vi "Cluster names.vi"(10 "Name":string, 11 "variant 2":variant) -> (0 "Array":variant[](array[variant]), 1 "Array 2":string[](array[string]), 2 "VCluster":variant, 3 "String":string)   [LabVIEW 2013]
uses:
  subVis/ROI_TypDef.ctl
  shared/OnOffTypeDef.ctl
  <vilib>/vision/Image Controls.llb/IMAQ Image.ctl
  <vilib>/userdefined/High Color/IMAQdx.ctl
  subVis/CamAtributes_TypDEfTestDevice.ctl
  subVis/TriggerModeString_TypDEf.ctl
  shared/numericVariable_TypeDef.ctl
  BaseDriver/BaseDriver.lvclass
panel:
  in  "Cluster of class private data":T7
  out "Data Name":string
  out "Array of VData":variant[](array[variant])
  in  "error in (no error)":errorcluster
  out "data out":string[][](array[string])
  in  "data in":string[][](array[string])=[["name", "value", "min", "max", "stepsize", "units", "variabletype", "tolerance", "valueactual"], ["Position.Axis 111", "0.000000000000000", "-999999", "999999", "0.000000000000000", "", "numeric", "0.000000000000000", "0.000000000000000"], ["Position.Axis 112", "0.000000000000000", "-999999", "999999", "0.000000000000000", "", "numeric", "0.000000000000000", "0.000000000000000"], ["Position.Axis 113", "0.000000000000000", "-999999", "999999", "0.000000000000000", "", "numeric", "0.000000000000000", "0.000000000000000"], ["Position.Axis 121", "0.000000000000000", "-999999", "999999", "0.000000000000000", "", "numeric", "0.000000000000000", "0.000000000000000"], ["Position.Axis 122", "0.000000000000000", "-999999", "999999", "0.000000000000000", "", "numeric", "0.000000000000000", "0.000000000000000"], ["Position.Axis 123", "0.000000000000000", "-999999", "999999", "0.000000000000000", "", "numeric", "0.000000000000000", "0.000000000000000"], ["Position.Axis 131", "0.000000000000000", "-999999", "999999", "0.000000000000000", "", "numeric", "0.000000000000000", "0.000000000000000"], ["Position.Axis 132", "0.000000000000000", "-999999", "999999", "0.000000000000000", "", "numeric", "0.000000000000000", "0.000000000000000"], ["Position.Axis 133", "0.000000000000000", "-999999", "999999", "0.000000000000000", "", "numeric", "0.000000000000000", "0.000000000000000"], ["Position.Axis 141", "0.000000000000000", "-999999", "999999", "0.000000000000000", "", "numeric", "0.000000000000000", "0.000000000000000"], ["Position.Axis 142", "0.000000000000000", "-999999", "999999", "0.000000000000000", "", "numeric", "0.000000000000000", "0.000000000000000"], ["Position.Axis 143", "0.000000000000000", "-999999", "999999", "0.000000000000000", "", "numeric", "0.000000000000000", "0.000000000000000"], ["Position.Axis 231", "0.000000000000000", "-999999", "999999", "0.000000000000000", "", "numeric", "0.000000000000000", "0.000000000000000"], ["Position.Axis 232", "0.000000000000000", "-999999", "-999999", "0.000000000000000", "", "numeric", "0.000000000000000", "0.000000000000000"], ["Position.Axis 233", "0.000000000000000", "-999999", "999999", "0.000000000000000", "", "numeric", "0.000000000000000", "0.000000000000000"], ["Position.Axis 241", "0.000000000000000", "-999999", "999999", "0.000000000000000", "", "numeric", "0.000000000000000", "0.000000000000000"], ["Position.Axis 242", "0.000000000000000", "-999999", "999999", "0.000000000000000", "", "numeric", "0.000000000000000", "0.000000000000000"], ["Position.Axis 243", "0.000000000000000", "-999999", "999999", "0.000000000000000", "", "numeric", "0.000000000000000", "0.000000000000000"], ["Position.Axis 311", "0.000000000000000", "-999999", "999999", "0.000000000000000", "", "numeric", "0.000000000000000", "0.000000000000000"], ["Position.Axis 312", "0.000000000000000", "-999999", "999999", "0.000000000000000", "", "numeric", "0.000000000000000", "0.000000000000000"], ["Position.Axis 321", "0.000000000000000", "-999999", "999999", "0.000000000000000", "", "numeric", "0.000000000000000", "0.000000000000000"], ["Position.Axis 322", "0.000000000000000", "-999999", "999999", "0.000000000000000", "", "numeric", "0.000000000000000", "0.000000000000000"], ["Position.Axis 323", "0.000000000000000", "-999999", "999999", "0.000000000000000", "", "numeric", "0.000000000000000", "0.000000000000000"], ["Position.Axis 331", "0.000000000000000", "-999999", "999999", "0.000000000000000", "", "numeric", "0.000000000000000", "0.000000000000000"], ["Position.Axis 332", "0.000000000000000", "-999999", "0.00000000000999999", "0.000000000000000", "", "numeric", "0.000000000000000", "0.000000000000000"], ["Position.Axis 333", "0.000000000000000", "-999999", "999999", "0.000000000000000", "", "numeric", "0.000000000000000", "0.000000000000000"], ["Position.Axis 341", "0.000000000000000", "-999999", "9999990000", "0.000000000000000", "", "numeric", "0.000000000000000", "0.000000000000000"], ["Position.Axis 342", "0.000000000000000", "-999999", "999999", "0.000000000000000", "", "numeric", "0.000000000000000", "0.000000000000000"], ["Position.Axis 343", "0.000000000000000", "-999999", "999999", "0.000000000000000", "", "numeric", "0.000000000000000", "0.000000000000000"], ["Position.Axis 411", "0.000000000000000", "-999999", "999999", "0.000000000000000", "", "numeric", "0.000000000000000", "0.000000000000000"], ["Position.Axis 412", "0.000000000000000", "-999999", "999999", "0.000000000000000", "", "numeric", "0.000000000000000", "0.000000000000000"], ["Position.Axis 413", "0.000000000000000", "-999999", "999999", "0.000000000000000", "", "numeric", "0.000000000000000", "0.000000000000000"], ["Position.Axis 421", "0.000000000000000", "-999999", "999999", "0.000000000000000", "", "numeric", "0.000000000000000", "0.000000000000000"], ["Position.Axis 422", "0.000000000000000", "-999999", "999999", "0.000000000000000", "", "numeric", "0.000000000000000", "0.000000000000000"], ["Position.Axis 423", "0.000000000000000", "-999999", "999999", "0.000000000000000", "", "numeric", "0.000000000000000", "0.000000000000000"], ["Position.Axis 431", "0.000000000000000", "-999999", "999999", "0.000000000000000", "", "numeric", "0.000000000000000", "0.000000000000000"], ["Position.Axis 432", "0.000000000000000", "-99999900000", "999999", "0.000000000000000", "", "numeric", "0.000000000000000", "0.000000000000000"], ["Position.Axis 433", "0.000000000000000", "-999999", "999999", "0.000000000000000", "", "numeric", "0.000000000000000", "0.000000000000000"], ["Position.Axis 441", "0.000000000000000", "-999999", "999999", "0.000000000000000", "", "numeric", "0.000000000000000", "0.000000000000000"], ["Position.Axis 442", "0.000000000000000", "-999999", "999999", "0.000000000000000", "", "numeric", "0.000000000000000", "0.000000000000000"], ["Position.Axis 443", "0.000000000000000", "-999999", "999999", "0.000000000000000", "", "numeric", "0.000000000000000", "0.000000000000000"], ["Position.Axis 511", "0.000000000000000", "-999999", "999999", "0.000000000000000", "", "numeric", "0.000000000000000", "0.000000000000000"], ["Position.Axis 512", "0.000000000000000", "-999999", "999999", "0.000000000000000", "", "numeric", "0.000000000000000", "0.000000000000000"], ["Position.Axis 513", "0.000000000000000", "-999999", "999999", "0.000000000000000", "", "numeric", "0.000000000000000", "0.000000000000000"], ["Position.Axis 521", "0.000000000000000", "-999999", "999999", "0.000000000000000", "", "numeric", "0.000000000000000", "0.000000000000000"], ["Position.Axis 522", "0.000000000000000", "-999999", "999999", "0.000000000000000", "", "numeric", "0.000000000000000", "0.000000000000000"], ["Position.Axis 523", "0.000000000000000", "-999999", "999999", "0.000000000000000", "", "numeric", "0.000000000000000", "0.000000000000000"], ["Position.Axis 531", "0.000000000000000", "-999999", "999999", "0.000000000000000", "", "numeric", "0.000000000000000", "0.000000000000000"], ["Position.Axis 532", "0.000000000000000", "-999999", "999999", "0.000000000000000", "", "numeric", "0.000000000000000", "0.000000000000000"], ["Position.Axis 533", "0.000000000000000", "-999999", "999999", "0.000000000000000", "", "numeric", "0.000000000000000", "0.000000000000000"], ["Position.Axis 541", "0.000000000000000", "-999999", "999999", "0.000000000000000", "", "numeric", "0.000000000000000", "0.000000000000000"], ["Position.Axis 542", "0.000000000000000", "-999999", "999999", "0.000000000000000", "", "numeric", "0.000000000000000", "0.000000000000000"], ["Position.Axis 543", "0.000000000000000", "-999999", "999999", "0.000000000000000", "", "numeric", "0.000000000000000", "0.000000000000000"], ["StepSize.Axis 111", "50", "0", "20000", "0.000000000000000", "", "numeric", "0.000000000000000", "0.000000000000000"], ["StepSize.Axis 112", "50", "0", "20000", "0.000000000000000", "", "numeric", "0.000000000000000", "0.000000000000000"], ["StepSize.Axis 113", "50", "0", "20000", "0.000000000000000", "", "numeric", "0.000000000000000", "0.000000000000000"], ["StepSize.Axis 121", "50", "0", "20000", "0.000000000000000", "", "numeric", "0.000000000000000", "0.000000000000000"], ["StepSize.Axis 122", "50", "0", "20000", "0.000000000000000", "", "numeric", "0.000000000000000", "0.000000000000000"], ["StepSize.Axis 123", "50", "0", "20000", "0.000000000000000", "", "numeric", "0.000000000000000", "0.000000000000000"], ["StepSize.Axis 131", "50", "0", "20000", "0.000000000000000", "", "numeric", "0.000000000000000", "0.000000000000000"], ["StepSize.Axis 132", "50", "0", "20000", "0.000000000000000", "", "numeric", "0.000000000000000", "0.000000000000000"], ["StepSize.Axis 133", "50", "0", "20000", "0.000000000000000", "", "numeric", "0.000000000000000", "0.000000000000000"], ["StepSize.Axis 141", "50", "0", "20000", "0.000000000000000", "", "numeric", "0.000000000000000", "0.000000000000000"], ["StepSize.Axis 142", "50", "0", "20000", "0.000000000000000", "", "numeric", "0.000000000000000", "0.000000000000000"], ["StepSize.Axis 143", "50", "0", "20000", "0.000000000000000", "", "numeric", "0.000000000000000", "0.000000000000000"], ["StepSize.Axis 211", "50", "0", "20000", "0.000000000000000", "", "numeric", "0.000000000000000", "0.000000000000000"], ["StepSize.Axis 212", "50", "0", "20000", "0.000000000000000", "", "numeric", "0.000000000000000", "0.000000000000000"], ["StepSize.Axis 213", "50", "0", "20000", "0.000000000000000", "", "numeric", "0.000000000000000", "0.000000000000000"], ["StepSize.Axis 231", "50", "0", "20000", "0.000000000000000", "", "numeric", "0.000000000000000", "0.000000000000000"], ["StepSize.Axis 232", "50", "0", "20000", "0.000000000000000", "", "numeric", "0.000000000000000", "0.000000000000000"], ["StepSize.Axis 233", "50", "0", "20000", "0.000000000000000", "", "numeric", "0.000000000000000", "0.000000000000000"], ["StepSize.Axis 241", "0", "0", "20000", "0.000000000000000", "", "numeric", "0.000000000000000", "0.000000000000000"], ["StepSize.Axis 242", "50", "0", "20000", "0.000000000000000", "", "numeric", "0.000000000000000", "0.000000000000000"], ["StepSize.Axis 243", "50", "0", "20000", "0.000000000000000", "", "numeric", "0.000000000000000", "0.000000000000000"], ["StepSize.Axis 311", "50", "0", "20000", "0.000000000000000", "", "numeric", "0.000000000000000", "0.000000000000000"], ["StepSize.Axis 312", "50", "0", "20000", "0.000000000000000", "", "numeric", "0.000000000000000", "0.000000000000000"], ["StepSize.Axis 321", "50", "0", "20000", "0.000000000000000", "", "numeric", "0.000000000000000", "0.000000000000000"], ["StepSize.Axis 322", "50", "0", "20000", "0.000000000000000", "", "numeric", "0.000000000000000", "0.000000000000000"], ["StepSize.Axis 323", "50", "0", "20000", "0.000000000000000", "", "numeric", "0.000000000000000", "0.000000000000000"], ["StepSize.Axis 331", "50", "0", "20000", "0.000000000000000", "", "numeric", "0.000000000000000", "0.000000000000000"], ["StepSize.Axis 332", "0", "0", "20000", "0.000000000000000", "", "numeric", "0.000000000000000", "0.000000000000000"], ["StepSize.Axis 333", "50", "0", "20000", "0.000000000000000", "", "numeric", "0.000000000000000", "0.000000000000000"], ["StepSize.Axis 341", "50", "0", "20000", "0.000000000000000", "", "numeric", "0.000000000000000", "0.000000000000000"], ["StepSize.Axis 342", "50", "0", "20000", "0.000000000000000", "", "numeric", "0.000000000000000", "0.000000000000000"], ["StepSize.Axis 343", "50", "0", "20000", "0.000000000000000", "", "numeric", "0.000000000000000", "0.000000000000000"], ["StepSize.Axis 411", "0", "0", "20000", "0.000000000000000", "", "numeric", "0.000000000000000", "0.000000000000000"], ["StepSize.Axis 412", "50", "0", "20000", "0.000000000000000", "", "numeric", "0.000000000000000", "0.000000000000000"], ["StepSize.Axis 413", "0", "0", "20000", "0.000000000000000", "", "numeric", "0.000000000000000", "0.000000000000000"], ["StepSize.Axis 421", "0", "0", "20000", "0.000000000000000", "", "numeric", "0.000000000000000", "0.000000000000000"], ["StepSize.Axis 422", "0", "0", "20000", "0.000000000000000", "", "numeric", "0.000000000000000", "0.000000000000000"], ["StepSize.Axis 423", "50", "0", "20000", "0.000000000000000", "", "numeric", "0.000000000000000", "0.000000000000000"], ["StepSize.Axis 431", "50", "0", "20000", "0.000000000000000", "", "numeric", "0.000000000000000", "0.000000000000000"], ["StepSize.Axis 432", "0", "0.00000000000", "20000", "0.000000000000000", "", "numeric", "0.000000000000000", "0.000000000000000"], ["StepSize.Axis 433", "0", "0", "20000", "0.000000000000000", "", "numeric", "0.000000000000000", "0.000000000000000"], ["StepSize.Axis 441", "0", "0", "20000", "0.000000000000000", "", "numeric", "0.000000000000000", "0.000000000000000"], ["StepSize.Axis 442", "0", "0.00000000000", "20000", "0.000000000000000", "", "numeric", "0.000000000000000", "0.000000000000000"], ["StepSize.Axis 443", "50", "0", "20000", "0.000000000000000", "", "numeric", "0.000000000000000", "0.000000000000000"], ["StepSize.Axis 511", "50", "0", "20000", "0.000000000000000", "", "numeric", "0.000000000000000", "0.000000000000000"], ["StepSize.Axis 512", "50", "0", "20000", "0.000000000000000", "", "numeric", "0.000000000000000", "0.000000000000000"], ["StepSize.Axis 513", "50", "0", "20000", "0.000000000000000", "", "numeric", "0.000000000000000", "0.000000000000000"], ["StepSize.Axis 521", "50", "0", "20000", "0.000000000000000", "", "numeric", "0.000000000000000", "0.000000000000000"], ["StepSize.Axis 522", "50", "0", "20000", "0.000000000000000", "", "numeric", "0.000000000000000", "0.000000000000000"], ["StepSize.Axis 523", "50", "000000", "20000", "0.000000000000000", "", "numeric", "0.000000000000000", "0.000000000000000"], ["StepSize.Axis 531", "50", "0", "20000", "0.000000000000000", "", "numeric", "0.000000000000000", "0.000000000000000"], ["StepSize.Axis 532", "50", "0", "20000", "0.000000000000000", "", "numeric", "0.000000000000000", "0.000000000000000"], ["StepSize.Axis 533", "50", "0", "20000", "0.000000000000000", "", "numeric", "0.000000000000000", "0.000000000000000"], ["StepSize.Axis 541", "50", "0", "20000", "0.000000000000000", "", "numeric", "0.000000000000000", "0.000000000000000"], ["StepSize.Axis 542", "50", "0", "20000", "0", "", "numeric", "0.000000000000000", "0.000000000000000"], ["StepSize.Axis 543", "50", "0", "200000", "0.000000000000000", "", "numeric", "0.000000000000000", "0.000000000000000"], ["ActiveMotorIndex", "", "", "", "", "", "string", "", ""], ["RelativeMove.Axis 1.CCW", "off", "", "", "", "", "on,off", "", ""], ["RelativeMove.Axis 1.CW", "off", "", "", "", "", "on,off", "", ""], ["RelativeMove.Axis 2.CCW", "off", "", "", "", "", "on,off", "", ""], ["RelativeMove.Axis 2.CW", "off", "", "", "", "", "on,off", "", ""], ["RelativeMove.Axis 3.CCW", "off", "", "", "", "", "on,off", "", ""], ["RelativeMove.Axis 3.CW", "off", "", "", "", "", "on,off", "", ""], ["Names.Motor 11", "PA2_Input1", "", "", "", "", "string", "", ""], ["Names.Motor 12", "PA2_Input2", "", "", "", "", "string", "", ""], ["Names.Motor 13", "L2_TelInpFar", "", "", "", "", "string", "", ""], ["Names.Motor 14", "L1_TelInpNear", "", "", "", "", "string", "", ""], ["Names.Motor 21", "", "", "", "", "", "string", "", ""], ["Names.Motor 24", "", "", "", "", "", "string", "", ""], ["Names.Motor 31", "", "", "", "", "", "string", "", ""], ["Names.Motor 32", "", "", "", "", "", "string", "", ""], ["Names.Motor 33", "", "", "", "", "", "string", "", ""], ["Names.Motor 34", "", "", "", "", "", "string", "", ""], ["Names.Motor 41", "", "", "", "", "", "string", "", ""], ["Names.Motor 42", "", "", "", "", "", "string", "", ""], ["Names.Motor 43", "", "", "", "", "", "string", "", ""], ["Names.Motor 44", "", "", "", "", "", "string", "", ""], ["Names.Motor 51", "", "", "", "", "", "string", "", ""], ["Names.Motor 52", "", "", "", "", "", "string", "", ""], ["Names.Motor 53", "", "", "", "", "", "string", "", ""], ["Names.Motor 54", "", "", "", "", "", "string", "", ""], ["RelativeSettings.Axis 1.StepSize", "0.000000000000000", "0.000000000000000", "999999", "0.000000000000000", "", "numeric", "0.000000000000000", "0.000000000000000"], ["RelativeSettings.Axis 2.Position", "0.000000000000000", "-999999", "999999", "0.000000000000000", "", "numeric", "0.000000000000000", "0.000000000000000"], ["RelativeSettings.Axis 2.StepSize", "0.000000000000000", "0.000000000000000", "999999", "0.000000000000000", "", "numeric", "0.000000000000000", "0.000000000000000"], ["RelativeSettings.Axis 3.Position", "0.000000000000000", "-9999990", "999999", "0.000000000000000", "", "numeric", "0.000000000000000", "0.000000000000000"], ["RelativeSettings.Axis 3.StepSize", "0.000000000000000", "0.000000000000000", "99999999", "0.000000000000000", "", "numeric", "0.000000000000000", "0.000000000000000"], ["Position.Axis 221", "10", "-20000", "20000", "0.000000000000000", "", "numeric", "0.000000000000000", "0.000000000000000"], ["VISAname", "GPIB0::9::INSTR", "", "", "", "", "string", "", ""], ["StepSize.Axis 222", "100", "0", "200000", "0.000000000000000", "", "numeric", "0.000000000000000", "0.000000000000000"], ["Position.Axis 222", "20", "-200000", "200000", "0.000000000000000", "", "numeric", "0.000000000000000", "0.000000000000000"], ["Names.Motor 22", "L5_TREXPass2", "", "", "", "", "string", "", ""], ["ActiveMotorName", "L5_TREXPass2", "", "", "", "", "string", "", ""], ["Names.Motor 23", "L6_TREXPass3", "", "", "", "", "string", "", ""], ["StepSize.Axis 221", "100", "-2000", "2000", "0.000000000000000", "", "numeric", "0.000000000000000", "0.000000000000000"], ["StepSize.Axis 223", "100", "0", "20000", "0.000000000000000", "", "numeric", "0.000000000000000", "0.000000000000000"], ["Position.Axis 212", "0", "-200000", "2000", "0.000000000000000", "", "numeric", "0.000000000000000", "0.000000000000000"], ["Position.Axis 213", "0", "-2000", "2000000", "0.000000000000000", "", "numeric", "0.000000000000000", "0.000000000000000"], ["Position.Axis 223", "0", "-20000", "200000000", "0.000000000000000", "", "numeric", "0.000000000000000", "0.000000000000000"], ["Position.Axis 211", "0.000000000000000", "-200000", "2000000", "0.000000000000000", "", "numeric", "0.000000000000000", "0.000000000000000"], ["RelativeSettings.Axis 1.Position", "0.000000000000000", "-999999", "999999", "0.000000000000000", "", "numeric", "0.000000000000000", "0.000000000000000"]]
  out "dataString":string
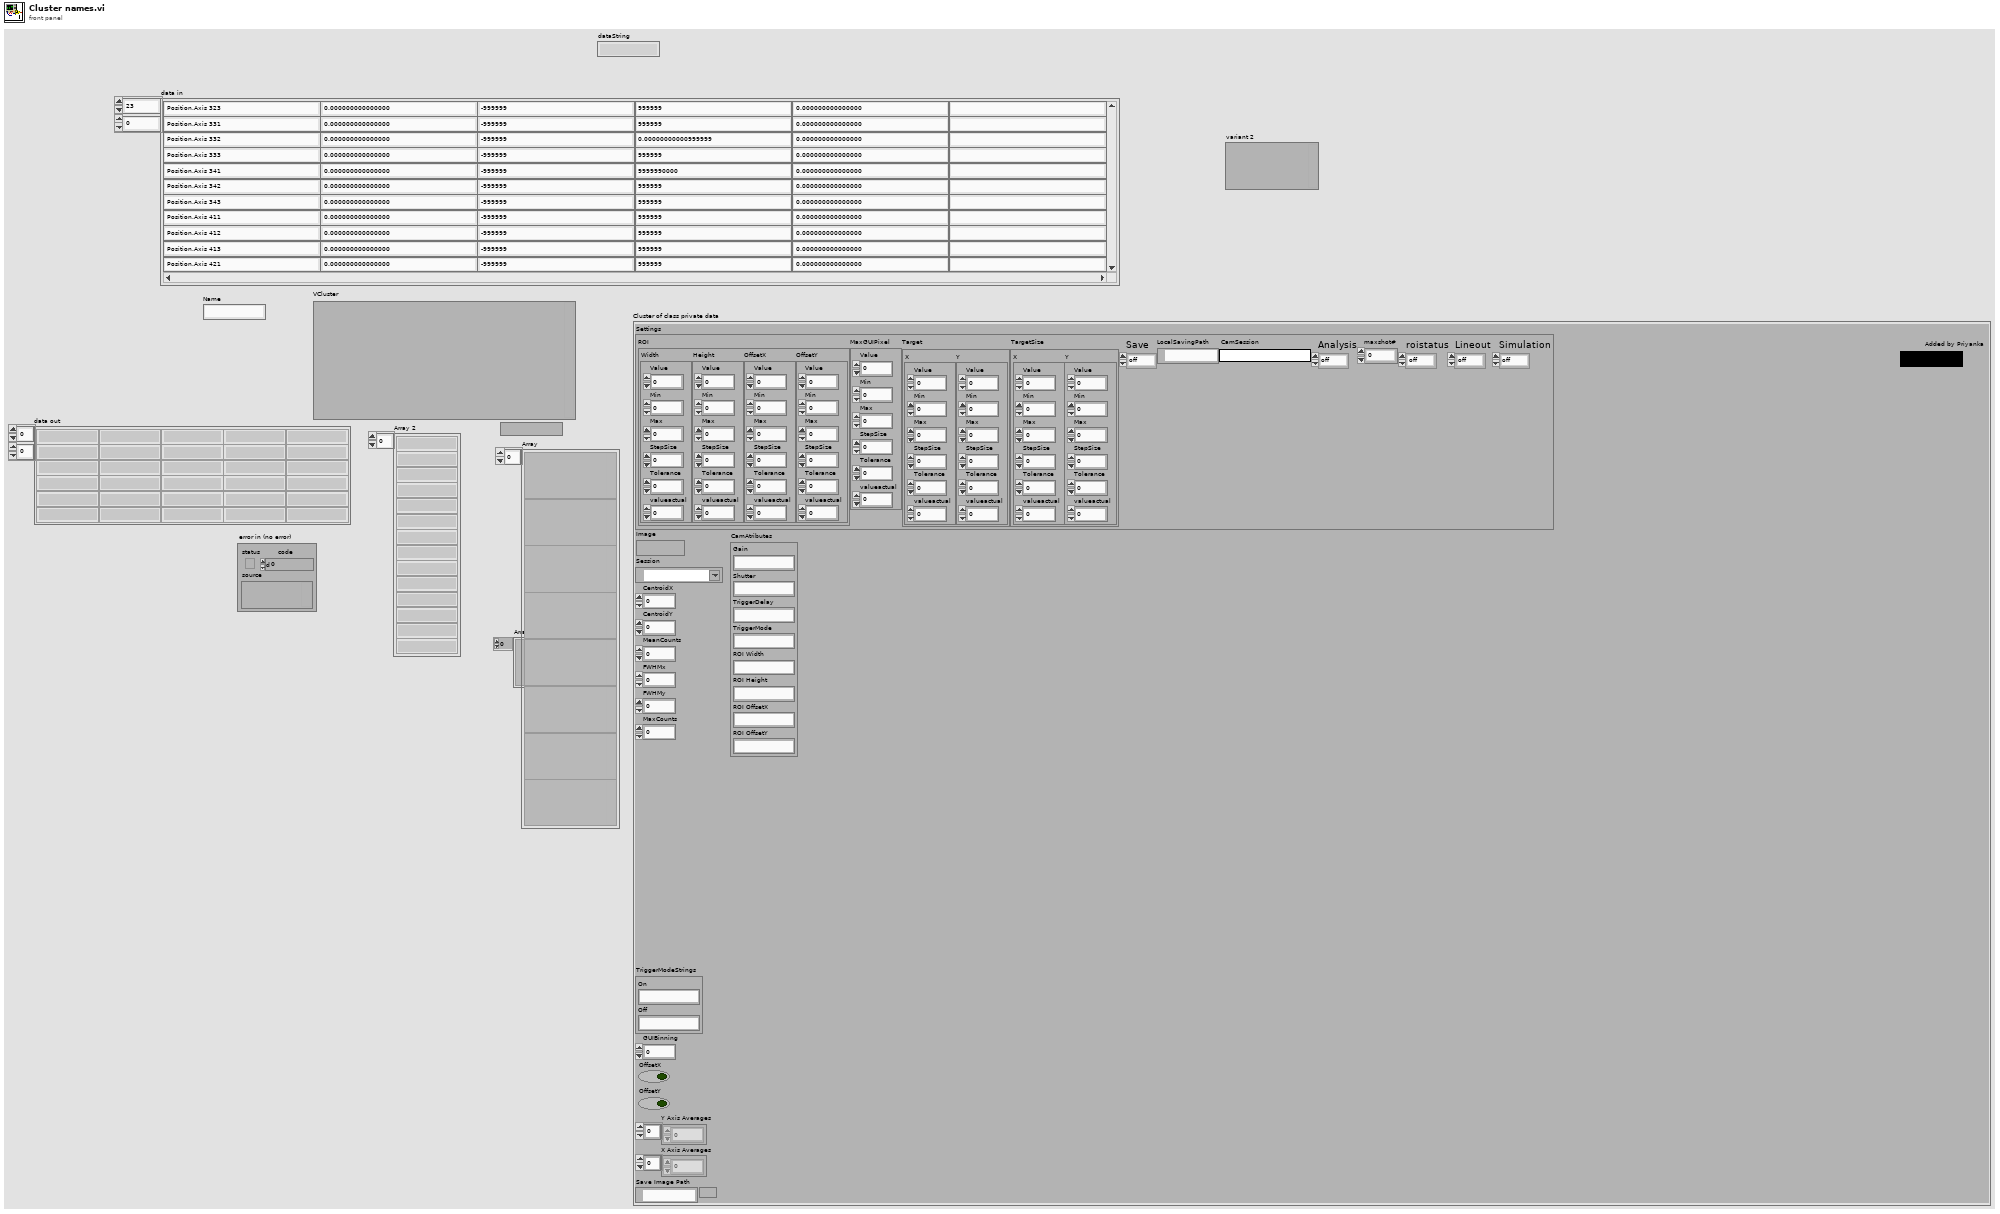
[diagram p1: front panel]
types:
  T1 = typedef "ROI_TypDef.ctl" = cluster{"Width":cluster{"Value":dbl, "Min":dbl, "Max":dbl, "StepSize":dbl, "Tolerance":dbl, "valueactual":dbl}, "Height":cluster{"Value":dbl, "Min":dbl, "Max":dbl, "StepSize":dbl, "Tolerance":dbl, "valueactual":dbl}, "OffsetX":cluster{"Value":dbl, "Min":dbl, "Max":dbl, "StepSize":dbl, "Tolerance":dbl, "valueactual":dbl}, "OffsetY":cluster{"Value":dbl, "Min":dbl, "Max":dbl, "StepSize":dbl, "Tolerance":dbl, "valueactual":dbl}}
  T2 = typedef "OnOffTypeDef.ctl" = enum16{"off", "on"}
  T3 = typedef "IMAQ Image.ctl" = refnum<image>
  T4 = typedef "IMAQdx.ctl" = refnum<k21>
  T5 = typedef "CamAtributes_TypDEfTestDevice.ctl" = cluster{"Gain":string, "Shutter":string, "TriggerDelay":string, "TriggerMode":string, "ROI Width":string, "ROI Height":string, "ROI OffsetX":string, "ROI OffsetY":string}
  T6 = typedef "TriggerModeString_TypDEf.ctl" = cluster{"On":string, "Off":string}
  T7 = cluster{"Settings":cluster{"ROI":T1, "MaxGUIPixel":cluster{"Value":dbl, "Min":dbl, "Max":dbl, "StepSize":dbl, "Tolerance":dbl, "valueactual":dbl}, "Target":cluster{"X":cluster{"Value":dbl, "Min":dbl, "Max":dbl, "StepSize":dbl, "Tolerance":dbl, "valueactual":dbl}, "Y":cluster{"Value":dbl, "Min":dbl, "Max":dbl, "StepSize":dbl, "Tolerance":dbl, "valueactual":dbl}}, "TargetSize":cluster{"X":cluster{"Value":dbl, "Min":dbl, "Max":dbl, "StepSize":dbl, "Tolerance":dbl, "valueactual":dbl}, "Y":cluster{"Value":dbl, "Min":dbl, "Max":dbl, "StepSize":dbl, "Tolerance":dbl, "valueactual":dbl}}, "Save":T2, "LocalSavingPath":path, "CamSession":string, "Analysis":T2, "maxshot#":dbl, "roistatus":T2, "Lineout":T2, "Simulation":T2}, "Image":T3, "Session":T4, "CentroidX":sgl, "CentroidY":sgl, "MeanCounts":sgl, "FWHMx":sgl, "FWHMy":sgl, "MaxCounts":sgl, "CamAtributes":T5, "TriggerModeStrings":T6, "GUIBinning":dbl, "OffsetX":bool, "OffsetY":bool, "Y Axis Averages":sgl[], "X Axis Averages":sgl[], "Save Image Path":path}
  T8 = typedef "BaseDriver.lvclass/numericVariable_TypeDef.ctl" = cluster{"Value":dbl, "Min":dbl, "Max":dbl, "StepSize":dbl, "Tolerance":dbl, "ValueActual":dbl}
  T9 = cluster{"ROI":T1, "MaxGUIPixel":cluster{"Value":dbl, "Min":dbl, "Max":dbl, "StepSize":dbl, "Tolerance":dbl, "valueactual":dbl}, "Target":cluster{"X":cluster{"Value":dbl, "Min":dbl, "Max":dbl, "StepSize":dbl, "Tolerance":dbl, "valueactual":dbl}, "Y":cluster{"Value":dbl, "Min":dbl, "Max":dbl, "StepSize":dbl, "Tolerance":dbl, "valueactual":dbl}}, "TargetSize":cluster{"X":cluster{"Value":dbl, "Min":dbl, "Max":dbl, "StepSize":dbl, "Tolerance":dbl, "valueactual":dbl}, "Y":cluster{"Value":dbl, "Min":dbl, "Max":dbl, "StepSize":dbl, "Tolerance":dbl, "valueactual":dbl}}, "Save":T2, "LocalSavingPath":path, "CamSession":string, "Analysis":T2, "maxshot#":dbl, "roistatus":T2, "Lineout":T2, "Simulation":T2}
  T10 = typedef "Type Descriptor Enumeration__ogtk.ctl" = enum8{"<Null>", "I8", "I16", "I32", "I64", "U8", "U16", "U32", "U64", "SGL", "DBL", "EXT", "CSG", "CDB", "CXT", "0x0F", "0x10", "0x11", "0x12", "0x13", "0x14", "Enum U8", "Enum U16", "Enum U32", "Enum U64", "SGL PQ", "DBL PQ", "EXT PQ", "CSG PQ", "CDB PQ", "CXT PQ", "0x1F", "0x20", "Boolean", "0x22", "0x23", "0x24", "0x25", "0x26", "0x27", "0x28", "0x29", "0x2A", "0x2B", "0x2C", "0x2D", "0x2E", "0x2F", "String", "0x31", "Path", "Pict", "0x34", "0x35", "0x36", "DAQ", "0x38", "0x39", "0x3A", "0x3B", "0x3C", "0x3D", "0x3E", "0x3F", "Array", "0x41", "0x42", "0x43", "0x44", "0x45", "0x46", "0x47", "0x48", "0x49", "0x4A", "0x4B", "0x4C", "0x4D", "0x4E", "0x4F", "Cluster", "0x51", "0x52", "Variant", "Waveform", "0x55", "0x56", "0x57", "0x58", "0x59", "0x5A", "0x5B", "0x5C", "0x5D", "0x5E", "0x5F", "0x60", "0x61", "0x62", "0x63", "0x64", "0x65", "0x66", "0x67", "0x68", "0x69", "0x6A", "0x6B", "0x6C", "0x6D", "0x6E", "0x6F", "Refnum"}
  T11 = typedef "Type Descriptor Header__ogtk.ctl" = cluster{"length":u16, "private":u8, "type":T10, "# elements":u16}
  T12 = typedef "Type Descriptor__ogtk.ctl" = i16[]
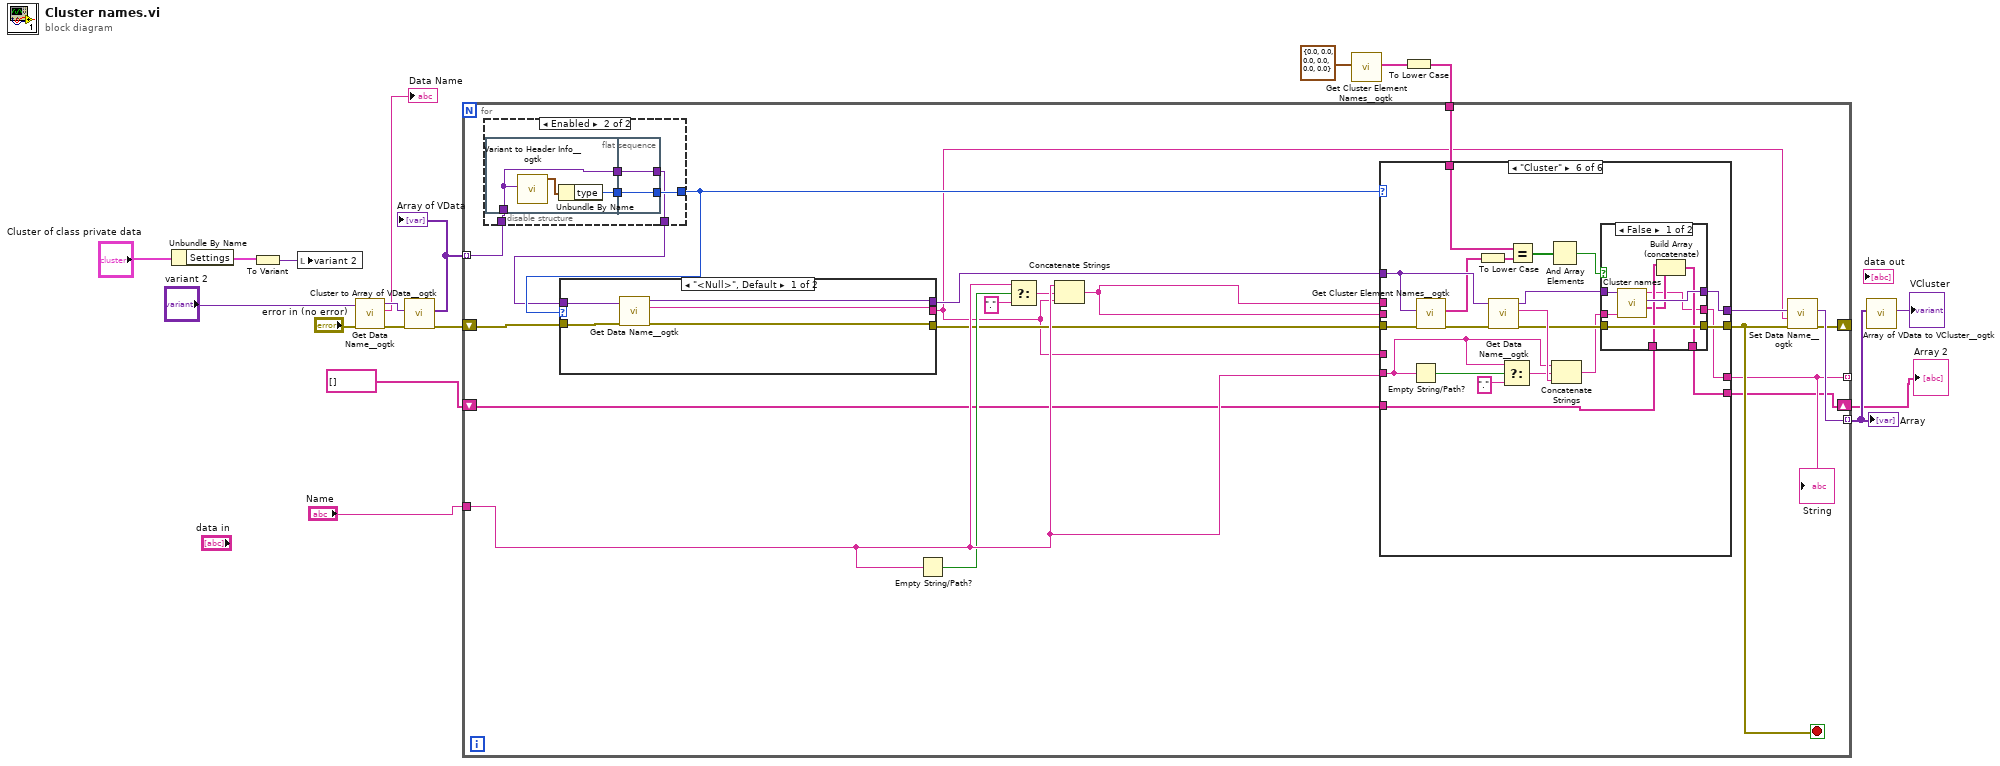
[diagram p0: block diagram]
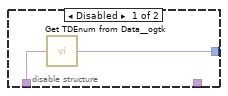
[diagram p2: hidden frame]
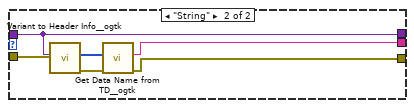
[diagram p3: hidden frame]
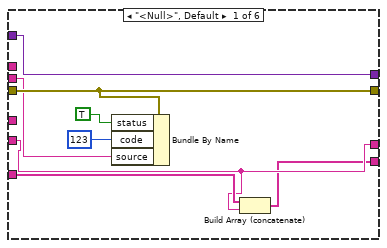
[diagram p4: hidden frame]
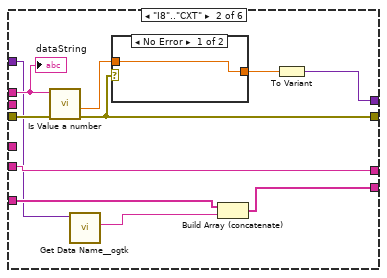
[diagram p5: hidden frame]
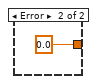
[diagram p6: hidden frame]
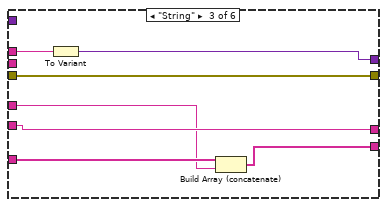
[diagram p7: hidden frame]
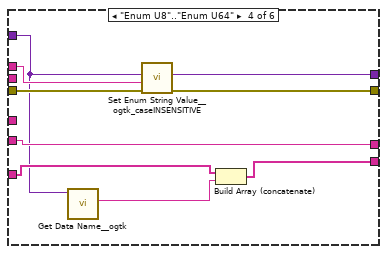
[diagram p8: hidden frame]
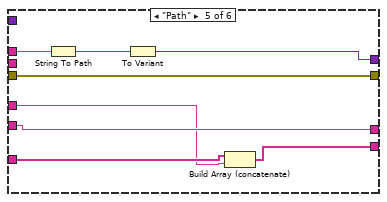
[diagram p9: hidden frame]
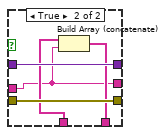
[diagram p10: hidden frame]
diagram:
  n1 = Unbundle By Name("Cluster of class private data") -> ("Settings"=w7:T9)
  n2 = To Variant(anything=w7) -> (Variant=w5:variant)
  n3 = local write "variant 2"(w5) -> ()
  n4 = call <userlib>:"Get Data Name__ogtk.vi"("error in (no error)"="error in (no error)", "Data"="variant 2") -> ("error out"=w13:errorcluster, "Data Name"=→"Data Name":string, "Data dup"=w17:variant)  [unwired: 7 in]
  n5 = call <userlib>:"Cluster to Array of VData__ogtk.vi"("error in (no error)"=w13, "Cluster"=w17) -> ("error out"=w12:errorcluster, "Array of VData"=w18:variant[])  [unwired: 8 in]
  "Array of VData" <- w18
  n6 = call <userlib>:"Get Cluster Element Names__ogtk.vi"("Cluster"=T8 {"Value"=0.0, "Min"=0.0, "Max"=0.0, "StepSize"=0.0, "Tolerance"=0.0, "ValueActual"=0.0} ("XXX")) -> ("Element Names"=w10:string[])  [unwired: 9 in, 1 out]
  n7 = To Lower Case(string=w10) -> (all lower case string=w9:string[])
  n8 = for {
    tunnel: w18 -> [w31] mode=indexing
    tunnel: "Name" -> [w36]
    shift-right: [w22] -> _
    shift-left: w12 -> [w37]
    tunnel: w9 -> [w33]
    tunnel: [w25] -> w4 mode=indexing
    tunnel: [w23] -> _ mode=indexing
    shift-right: [w20] -> w1
    shift-left: string[] [] -> [w21]
    stop <- w27 stop-if-true
    n9 = disable-structure shown="Enabled" {
      disable-tunnel: w31 -> [w40 w45]
      disable-tunnel: [w39 w44] -> w30
      disable-tunnel: [_ w41] -> w29
      frame Disabled {
        n10 = call <userlib>:"Get TDEnum from Data__ogtk.vi"("Data"=w40) -> ("Type Descriptor Enumeration"=w39:T10)  [unwired: 4 in]
      }
      frame Enabled {
        n11 = flat-sequence {
          tunnel: w45 -> [w46]
          tunnel: [w47] -> w43
          tunnel: [w46] -> w42
          tunnel: [w50] -> w44
          tunnel: w43 -> [w50]
          tunnel: w42 -> [w49]
          tunnel: [w49] -> w41
          frame #0 {
            n12 = call <userlib>:"Variant to Header Info__ogtk.vi"("Variant"=w46) -> ("Type Descriptor Header"=w48:T11)  [unwired: 3 in, 2 out]
            n13 = Unbundle By Name(w48) -> ("type"=w47:T10)
          }
          frame #1 {
          }
        }
      }
    }
    n14 = case shown="\"<Null>\", Default" w30 {
      tunnel: w37 -> [w54 w60]
      tunnel: [w53 w59] -> w26
      tunnel: w29 -> [w55 w56]
      tunnel: [w52 w57] -> w19
      tunnel: [w51 w56] -> w28
      frame "<Null>", Default {
        n15 = call <userlib>:"Get Data Name__ogtk.vi"("error in (no error)"=w54, "Data"=w55) -> ("error out"=w53:errorcluster, "Data Name"=w52:string, "Data dup"=w51:variant)  [unwired: 7 in]
      }
      frame "String" {
        n16 = call <userlib>:"Variant to Header Info__ogtk.vi"("Variant"=w56) -> ("Type Descriptor"=w58:T12)  [unwired: 3 in, 2 out]
        n17 = call <userlib>:"Get Data Name from TD__ogtk.vi"("error in (no error)"=w60, "Type Descriptor"=w58) -> ("error"=w59:errorcluster, "name"=w57:string)  [unwired: 8 in]
      }
    }
    n18 = Empty String/Path?(string/path=w36) -> (empty?=w32:bool)
    n19 = Select(t=w36, s=w32, f="." ("string")) -> (s? t:f=w34:string)
    n20 = Concatenate Strings(w36, w34, w19) -> (w24:string)
    n21 = case shown="\"Cluster\"" w30 {
      tunnel: w28 -> [w68 w70 _ w90 _ w124]
      tunnel: [w68 w79 w88 w95 w104 w110] -> w38
      tunnel: w36 -> [w62 w73 w85 w93 w101 w121]
      tunnel: w24 -> [_ w71 w83 w91 w99 _]
      tunnel: w26 -> [w67 w76 w87 w97 w103 w118]
      tunnel: [w67 w75 w87 w96 w103 w115] -> w27
      tunnel: w24 -> [w64 _ _ _ _ _]
      tunnel: w33 -> [_ _ _ _ _ w114]
      tunnel: [w62 w73 w85 w93 w101 w108] -> w23
      tunnel: w21 -> [w63 w74 w86 w94 w102 w107]
      tunnel: [w61 w72 w84 w92 w100 w106] -> w20
      tunnel: w19 -> [_ _ w82 _ w98 _]
      frame "<Null>", Default {
        n22 = Bundle By Name(cluster=w67, "status"=TRUE, "code"=123, "source"=w64) -> ()  [unwired: 1 out]
        n23 = Build Array (concatenate)(w63, w62) -> (w61:string[])
      }
      frame "I8".."CXT" {
        n24 = call "Is Value a number.vi"("user error in"=w76, "value String"=w71) -> ("user error out"=w75:errorcluster, "number"=w78:dbl)  [unwired: 6 in, 2 out]
        n25 = call <userlib>:"Get Data Name__ogtk.vi"("Data"=w70) -> ("Data Name"=w69:string)  [unwired: 8 in, 2 out]
        n26 = case shown="No Error" w75 {
          tunnel: w78 -> [w80 _]
          tunnel: [w80 0.0 ("number")] -> w77
          frame No Error {
          }
          frame Error {
          }
        }
        n27 = Build Array (concatenate)(w74, w69) -> (w72:string[])
        n28 = To Variant(anything=w77) -> (Variant=w79:variant)
        "dataString" <- w71
      }
      frame "String" {
        n29 = To Variant(anything=w83) -> (Variant=w88:variant)
        n30 = Build Array (concatenate)(w86, w82) -> (w84:string[])
      }
      frame "Enum U8".."Enum U64" {
        n31 = call <userlib>:"Get Data Name__ogtk.vi"("Data"=w90) -> ("Data Name"=w89:string)  [unwired: 8 in, 2 out]
        n32 = call "Set Enum String Value__ogtk_caseINSENSITIVE.vi"("error in (no error)"=w97, "String Value"=w91, "Default Enum Value"=w90) -> ("error out"=w96:errorcluster, "Enum"=w95:variant)  [unwired: 7 in]
        n33 = Build Array (concatenate)(w94, w89) -> (w92:string[])
      }
      frame "Path" {
        n34 = String To Path(string=w99) -> (path=w105:path)
        n35 = To Variant(anything=w105) -> (Variant=w104:variant)
        n36 = Build Array (concatenate)(w102, w98) -> (w100:string[])
      }
      frame "Cluster" {
        n37 = Empty String/Path?(string/path=w121) -> (empty?=w122:bool)
        n38 = call <userlib>:"Get Cluster Element Names__ogtk.vi"("error in (no error)"=w118, "Cluster"=w124) -> ("error out"=w117:errorcluster, "Element Names"=w113:string[])  [unwired: 8 in]
        n39 = To Lower Case(string=w113) -> (all lower case string=w112:string[])
        n40 = call <userlib>:"Get Data Name__ogtk.vi"("error in (no error)"=w117, "Data"=w124) -> ("error out"=w116:errorcluster, "Data Name"=w123:string, "Data dup"=w111:variant)  [unwired: 7 in]
        n41 = Select(t=w121, s=w122, f="." ("string")) -> (s? t:f=w119:string)
        n42 = Equal?(x=w114, y=w112) -> (x = y?=w126:bool[])
        n43 = And Array Elements(Boolean array=w126) -> (logical AND=w125:bool)
        n44 = Concatenate Strings(w121, w119, w123) -> (w109:string)
        n45 = case shown="False" w125 {
          tunnel: w111 -> [w133 w138]
          tunnel: w109 -> [w132 w135]
          tunnel: w116 -> [w134 w139]
          tunnel: [w134 w139] -> w115
          tunnel: [w131 w138] -> w110
          tunnel: [w127 w135] -> w108
          tunnel: w107 -> [w130 w137]
          tunnel: [w129 w136] -> w106
          frame False {
            n46 = call "Cluster names.vi"("Name"=w132, "variant 2"=w133) -> ("Array 2"=w128:string[], "VCluster"=w131:variant, "String"=w127:string)  [unwired: 6 in, 1 out]
            n47 = Build Array (concatenate)(w130, w128) -> (w129:string[])
          }
          frame True {
            n48 = Build Array (concatenate)(w137, w135) -> (w136:string[])
          }
        }
      }
    }
    "String" <- w23
    n49 = call <userlib>:"Set Data Name__ogtk.vi"("error in (no error)"=w27, "Data Name"=w19, "Data"=w38) -> ("error out"=w22:errorcluster, "Renamed Data"=w25:variant)  [unwired: 7 in]
  }
  "Array" <- w4
  "Array 2" <- w1
  n50 = call <userlib>:"Array of VData to VCluster__ogtk.vi"("Array"=w4) -> ("VCluster"=→"VCluster":variant)  [unwired: 9 in, 1 out]
